vi "Shutdown.vi"(8 "error in (no error)":errorcluster, 9 "wait timeout in ms (-1)":i32=-1, 10 "Wait until shutdown? (F)":bool, 11 "BluePlotHandle in":refnum<class "BluePlotHandle.lvclass">) -> (0 "error out":errorcluster)   [LabVIEW 2021, in "BluePlot.lvlib" / "BluePlotHandle.lvclass"]
uses:
  BluePlotHandle.lvclass
  BluePlotHandle.lvclass/BluePlotHandle.ctl
  TypeDefs/plot handle queue data.ctl
  TypeDefs/Plot QSM action.ctl
  <vilib>/Utility/error.llb/Clear Errors.vi
  BluePlot.lvlib
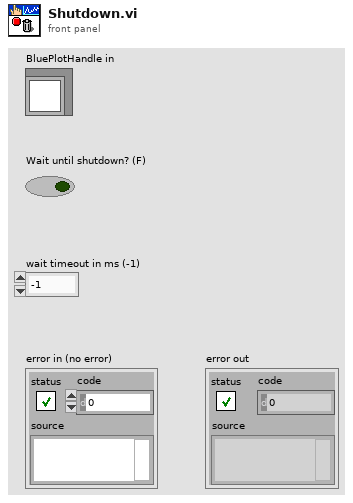
[diagram p1: front panel]
types:
  T1 = typedef "BluePlot.lvlib/Plot QSM action.ctl" = enum16{"start updating", "stop updating", "Shutdown", "Update", "Init", "Get Config", "Load Config"}
  T2 = typedef "BluePlot.lvlib/plot handle queue data.ctl" = cluster{"action":T1, "data":variant}
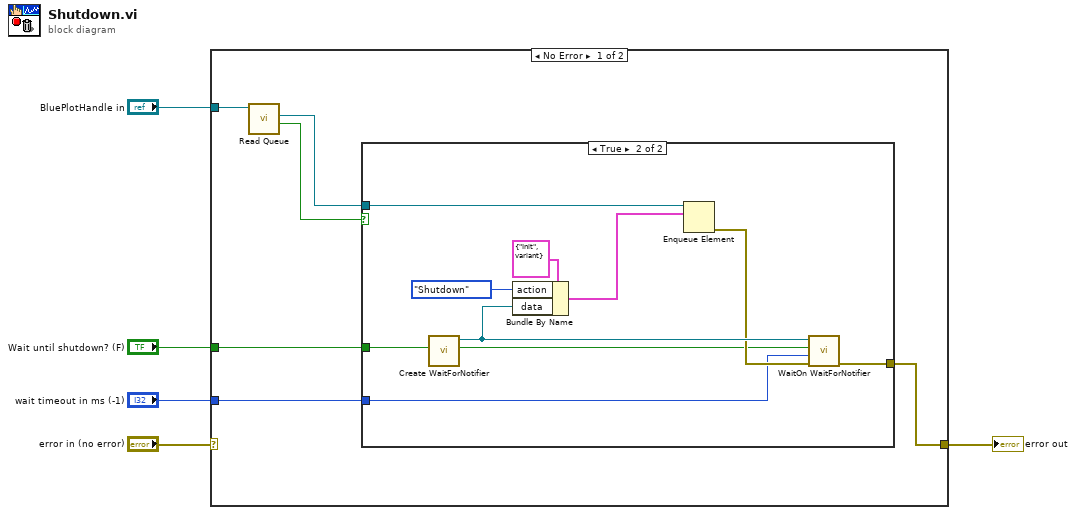
[diagram p0: block diagram]
diagram:
  n1 = case shown="No Error" "error in (no error)" {
    selector: "error in (no error)" -> [_ w22]
    tunnel: "BluePlotHandle in" -> [w10 _]
    tunnel: "Wait until shutdown? (F)" -> [w8 _]
    tunnel: "wait timeout in ms (-1)" -> [w7 _]
    tunnel: [w6 w22] -> w1
    frame No Error {
      n2 = call "Read Queue.vi"("BluePlotHandle in"=w10) -> ("Valid?"=w11:bool, "Queue"=w9:refnum<queue>)  [unwired: 8 in, 1 out]
      n3 = case shown="True" w11 {
        tunnel: w9 -> [_ w21]
        tunnel: w8 -> [_ w17]
        tunnel: w7 -> [_ w13]
        tunnel: [_ w12] -> w6
        frame False {
        }
        frame True {
          n4 = call "Create WaitForNotifier.vi"("Wait until finished?"=w17) -> ("Wait until finished? (dup)"=w14:bool, "notifier"=w16:refnum<notifier>)  [unwired: 9 in]
          n5 = Bundle By Name(cluster=T2 {"action"=enum."Init", "data"=variant} ("element"), "action"=Plot_QSM_action."Shutdown", "data"=w16) -> (w18:T2)
          n6 = Enqueue Element(queue=w21, element=w18) -> (error out=w15:errorcluster)  [unwired: 2 in, 2 out]
          n7 = call "WaitOn WaitForNotifier.vi"("error in (no error)"=w15, "timeout in ms (-1)"=w13, "Wait until finished?"=w14, "notifier"=w16) -> ("error out"=w12:errorcluster)  [unwired: 6 in, 1 out]
        }
      }
    }
    frame Error {
    }
  }
  "error out" <- w1
